vi "nav1.vi"(9 "Drone":T3, 11 "Field":T1[][](array[typedef])) -> (2 "Move?":bool, 3 "direction":T2 items=["^", "^>", ">", "V>", "V", "<V", "<", "<^"])   [LabVIEW 2009]
uses:
  Drone data.ctl
  direction.ctl
  square.ctl
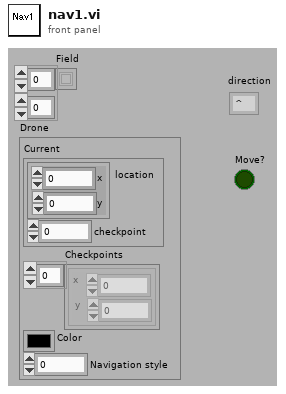
[diagram p1: front panel]
types:
  T1 = typedef "square.ctl" = u8
  T2 = typedef "direction.ctl" = i8
  T3 = typedef "Drone data.ctl" = cluster{"Current":cluster{"location":cluster{"x":i16, "y":i16}, "checkpoint":i32}, "Checkpoints":cluster{"x":i16, "y":i16}[], "Color":u32, "Navigation style":i32}
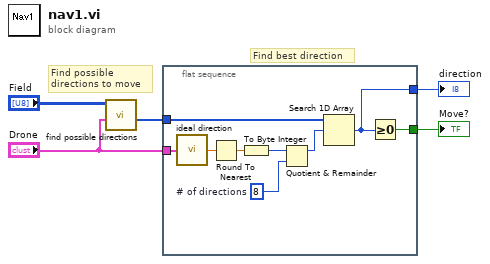
[diagram p0: block diagram]
diagram:
  # "Find possible\ndirections to move"
  # "Find best direction"
  n1 = call "find possible directions.vi"("Drone"="Drone", "Field"="Field") -> ("possible directions"=w3:T2[])  [unwired: 8 in, 1 out]
  n2 = flat-sequence {
    tunnel: "Drone" -> [w14]
    tunnel: w3 -> [w10]
    tunnel: [w7] -> w5
    tunnel: [w6] -> w4
    frame #0 {
      w12 = i8 8  # # of directions
      n3 = call "ideal direction.vi"("Drone"=w14) -> ("ideal direction"=w13:dbl)
      n4 = Round To Nearest(number=w13) -> (nearest integer value=w11:dbl)
      n5 = To Byte Integer(number=w11) -> (8bit integer=w8:i8)
      n6 = Quotient & Remainder(x=w8, y=w12) -> (x-y*floor(x/y)=w9:i8)  [unwired: 1 out]
      n7 = Search 1D Array(1D array=w10, element=w9) -> (index of element=w7:i32)  [unwired: 1 in]
      n8 = Greater Or Equal To 0?(x=w7) -> (x >= 0?=w6:bool)
    }
  }
  "direction" <- w5
  "Move?" <- w4
